vi "Configure Digital Pattern Frequency.vi"(8 "error in (no error)":errorcluster, 10 "Frequency (1000 Hz)":dbl=1000.0 min=1e-06 max=50000000.0, 11 "VISA resource name":refnum<visa-resource-name>) -> (0 "error out":errorcluster, 3 "VISA resource name out":refnum<visa-resource-name>)   [LabVIEW 2017, in "Keithley 3390.lvlib"]
doc: "Changes the frequency of the digital pattern output."
uses:
  Keithley 3390.lvlib
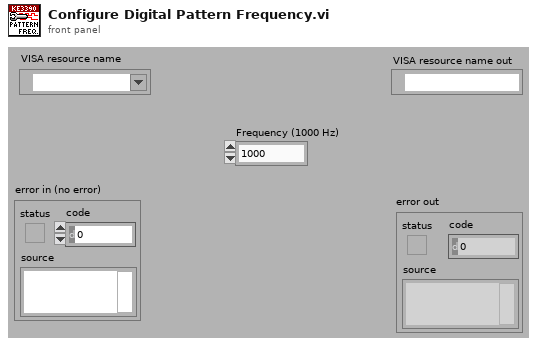
[diagram p1: front panel]
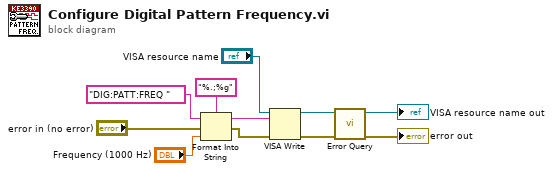
[diagram p0: block diagram]
diagram:
  n1 = Format Into String(format string="%.;%g", initial string="DIG:PATT:FREQ " ("command"), error in="error in (no error)", "Frequency (1000 Hz)") -> (resulting string=w7:string, error out=w8:errorcluster)
  n2 = VISA Write(VISA resource name="VISA resource name", write buffer=w7, error in (no error)=w8) -> (VISA resource name out=w4:refnum<visa-resource-name>, error out=w3:errorcluster)  [unwired: 1 out]
  n3 = call "Error Query.vi"("error in (no error)"=w3, "VISA resource name"=w4) -> ("error out"=→"error out":errorcluster, "VISA resource name out"=→"VISA resource name out":refnum<visa-resource-name>)  [unwired: 6 in, 2 out]
